vi "Test_Flip_Flop.vi"() -> ()   [LabVIEW 2022 SP3]
panel:
  out "BO1":bool
  out "BO2":bool
  in  "BI1":bool
  in  "BI2":bool
  in  "stop":bool
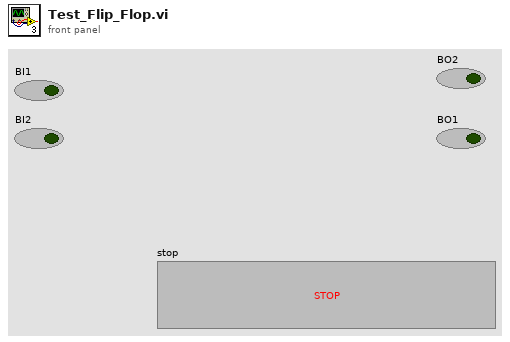
[diagram p1: front panel]
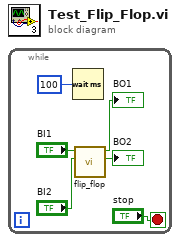
[diagram p0: block diagram]
diagram:
  n1 = while {
    stop <- "stop" stop-if-true
    n2 = Wait (ms)(milliseconds to wait=u32 100) -> ()  [unwired: 1 out]
    n3 = call "flip_flop.vi"("BI2"="BI2", "BI1"="BI1") -> ("BO2"=→"BO2":bool, "BO1"=→"BO1":bool)  [unwired: 7 in, 1 out]
  }
